vi "setTriggerSource.vi"(8 "error in (no error)":errorcluster, 10 "Source":enum16{"Immediate", "External", "Timer", "Bus"}(ring), 11 "VISA resource name":refnum<visa-resource-name>) -> (0 "error out":errorcluster, 3 "VISA resource name out":refnum<visa-resource-name>)   [LabVIEW 2023, in "Keysight-33500B.lvlib"]
doc: "<b>Author:</b> Wolfgang\n<b>Description:</b>\n<b>IMMediate (internal)</b>: the instrument outputs continuously when burst mode is enabled. The rate at which the burst is generated is determined by BURSt:INTernal:PERiod.\n<b>EXTernal</b>: the instrument accepts a hardware trigger at the rear-panel Ext Trig connector. The instrument outputs one burst of the specified number of cycles each time Ext Trig receives a level transition with the proper polarity (TRIGger[1|2]:SLOPe). External trigger signals during a burst are ignored.\n<b>BUS (software)</b>: the instrument initiates one burst each time a bus trigger (*TRG) is received. The front panel [Trigger] key is illuminated when the instrument is waiting for a bus trigger. \n<b>EXTernal or BUS</b>: burst count and burst phase remain in effect, but burst period is ignored.\n<b>TIMer:</b> trigger events are spaced by a timer, with the first trigger as soon as INIT occurs."
uses:
  Keysight-33500B.lvlib
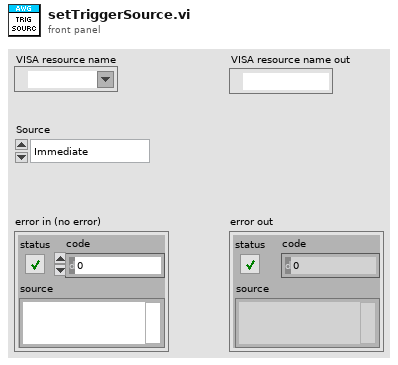
[diagram p1: front panel]
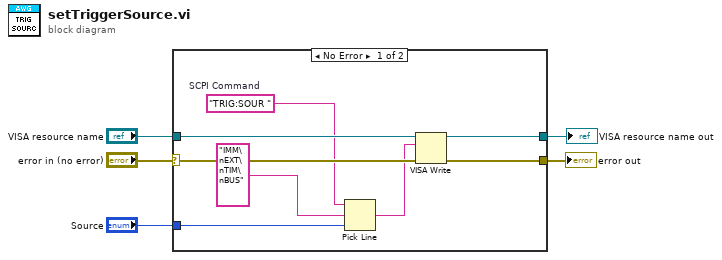
[diagram p0: block diagram]
diagram:
  n1 = case shown="No Error" "error in (no error)" {
    selector: "error in (no error)" -> [w10 w15]
    tunnel: [w12 w14] -> w5
    tunnel: [w13 w15] -> w3
    tunnel: "VISA resource name" -> [w11 w14]
    tunnel: "Source" -> [w9 _]
    frame No Error {
      w8 = "TRIG:SOUR "  # SCPI Command
      n2 = Pick Line(string ("")=w8, multi-line string="IMM\nEXT\nTIM\nBUS", line index=w9) -> (output string=w7:string)
      n3 = VISA Write(VISA resource name=w11, write buffer=w7, error in (no error)=w10) -> (VISA resource name out=w12:refnum<visa-resource-name>, error out=w13:errorcluster)  [unwired: 1 out]
    }
    frame Error {
    }
  }
  "VISA resource name out" <- w5
  "error out" <- w3
